vi "N1.vi"   [LabVIEW 2013]
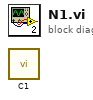
[diagram p0: block diagram]
diagram:
  n1 = call "C1.vi"() -> ()  [unwired: 7 in, 5 out]
